vi "Init Events.vi"(8 "error in (no error)":errorcluster, 11 "Main in":refnum<class "Main.lvclass">) -> (0 "error out":errorcluster, 3 "Main out":refnum<class "Main.lvclass">)   [LabVIEW 2019, in "Main.lvclass"]
doc: "Developed by Kevin Thompson\nkevin@thompsonengineering.net\n\nCopyright 2018\nThompson Engineering, LLC"
uses:
  Main.lvclass
  Common/DataTypes/TD Async CmdMsg EventData--cluster.ctl
  Common/DataTypes/UpdateControlValue EvData--cluster.ctl
  DataTypes/ProcessingState--enum.ctl
  DataTypes/ProcessingStateChg EvData--cluster.ctl
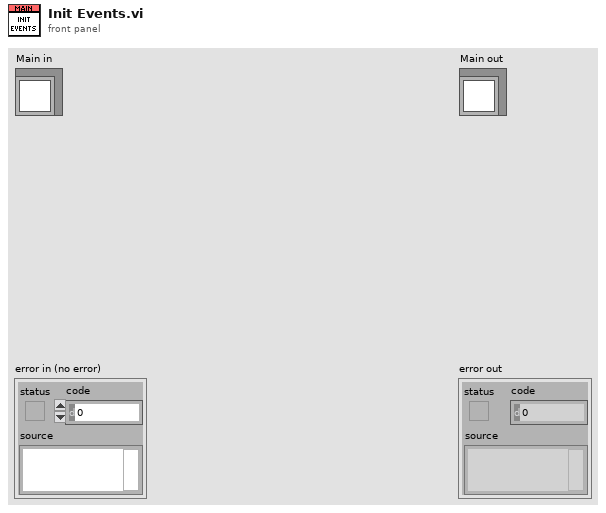
[diagram p1: front panel]
types:
  T1 = typedef "Main.lvclass/ProcessingStateChg EvData--cluster.ctl" = cluster{"Time Stamp":timestamp, "OLD ProcessingState":T2, "NEW ProcessingState":T2}
  T2 = typedef "Main.lvclass/ProcessingState--enum.ctl" = enum16{"Idle", "Starting", "Running", "Done", "Error"}
  T3 = typedef "UpdateControlValue EvData--cluster.ctl" = cluster{"Time Stamp":timestamp, "ControlLabel":string, "vData":variant}
  T4 = typedef "TD Async CmdMsg EventData--cluster.ctl" = cluster{"Time Stamp":timestamp, "CmdMsg":string, "vData":variant}
  T5 = typedef "Main.lvclass/Public Events--cluster.ctl" = cluster{"Main.AsyncCmd Event":refnum<user-event>, "Main.AsyncMsg Event":refnum<user-event>, "stop process":refnum<user-event>, "UpdateControlValue Ev":refnum<user-event>, "ProcessingStateChg Ev":refnum<user-event>}
  T6 = typedef "Main.lvclass/ObjData--cluster.ctl" = cluster{"Settings":T7, "Public Events":T5, "Dependency":T10, "ReadData-placeholder":T11, "VISA-placeholder":refnum<visa-resource-name>, "InverterWaveformsQ":T12, "Application.TerminateProcess Event":refnum<user-event>, "RawDaqDataQ":T13, "MeasSettings":T14, "InverterDataAcqMode":T15, "DAQState Data":T16, "Private Events":T18, "InvWfmsQ-DT":T12, "DPAuxDataQ":T19, "ProcessingState":T2, "InverterInfo":T20, "CurrInverters":T21[], "InverterLUT Dict":T25, "ESR Chart Ref":refnum<vi>, "StoreESR BLine Ref":refnum<vi>, "UseSavedESR BLine Ref":refnum<vi>}
  T7 = typedef "Main.lvclass/Settings--cluster.ctl" = cluster{"Simulation":bool, "Signal scaling":T8[], "ESR scaling":T9[], "num readings to average":i32[], "ESR alarm threshhold (%)":i32[], "UseDummyVrms":bool, "Dummy Vrms":dbl, "Inverter Database File":path, "default Inverter (name)":string[]}
  T8 = typedef "Main.lvclass/Gain control.ctl" = cluster{"Iin ripple gain":dbl, "Iout ripple gain":dbl, "Iout 60Hz gain ":dbl, "Vout 60Hz gain ":dbl, "Iin ripple offest":dbl, "Iout ripple offset":dbl, "Iout 60Hz offset":dbl, "Vout 60Hz offset":dbl}
  T9 = typedef "Main.lvclass/ESR scaling--cluster.ctl" = cluster{"Gain":dbl, "Offset":dbl}
  T10 = typedef "Main.lvclass/Dependency--cluster.ctl" = cluster{"Config":refnum<class "Config.lvclass">, "DAQ":refnum<class "DAQ_Engine.lvclass">, "Log_Engine":refnum<class "Log_Engine.lvclass">}
  T11 = typedef "Main.lvclass/Read Data--cluster.ctl" = cluster{"Data":dbl}
  T12 = typedef "InverterWaveforms--QRef.ctl" = refnum<queue>
  T13 = typedef "RawDAQDataQRef--cluster.ctl" = refnum<queue>
  T14 = typedef "Measurement Config--cluster.ctl" = cluster{"Data Rate 9775":dbl, "Data Rate 9215":dbl, "Samples RMS 9215":u32, "Samples RMS 9775":u32}
  T15 = typedef "Acquisition Mode--cluster.ctl" = enum16{"3phase", "Single"}
  T16 = typedef "DAQ_Engine.lvclass/DAQStateEvData--cluster.ctl" = cluster{"DAQState":T17, "vData":variant}
  T17 = typedef "DAQState--enum.ctl" = enum16{"Unknown", "Stopped", "Running", "Error"}
  T18 = typedef "Main.lvclass/Private Events--cluster.ctl" = cluster{"PrivateAsync Ev":refnum<user-event>}
  T19 = typedef "DataProcAuxDat--Qref.ctl" = refnum<queue>
  T20 = typedef "InverterInfo--cluster.ctl" = cluster{"Inverter ID":string}
  T21 = typedef "Inverter database record v2--cluster.ctl" = cluster{"name":string, "last updated":timestamp, "type":string, "inverter Info":T22, "gain range":T23, "offset range":T24, "gain actual":dbl, "offset actual":dbl, "power level":dbl, "minimum current":dbl, "resistance single phase":dbl, "resistance 3 phase":dbl, "set flag":u16}
  T22 = typedef "inverter info v2--cluster.ctl" = cluster{"manufacturer":string, "model":string, "product":string, "serial":string, "power class":string, "year manf":string}
  T23 = typedef "inverter gain range--cluster.ctl" = cluster{"gain max":dbl, "gain min":dbl, "gain increment":dbl}
  T24 = typedef "inverter offset range--cluster.ctl" = cluster{"offset max":dbl, "offset min":dbl, "offset increment":dbl}
  T25 = typedef "TD Dynamic CVT DVR--ref.ctl" = refnum<data-value>
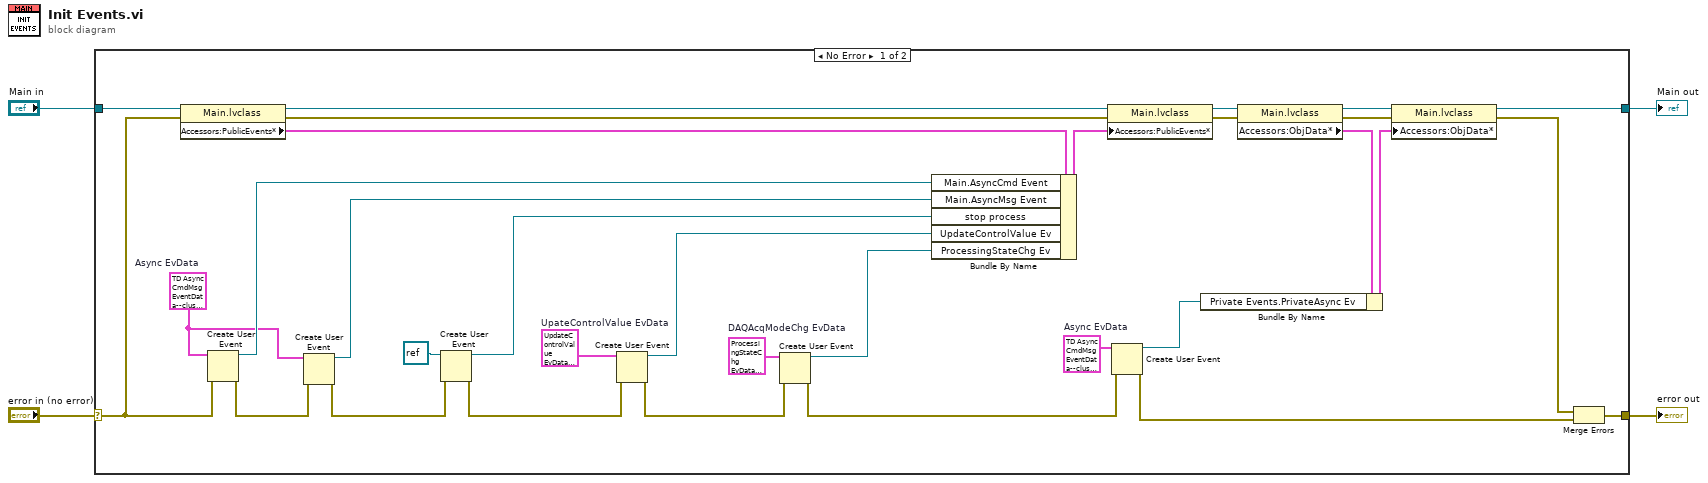
[diagram p0: block diagram]
diagram:
  n1 = case shown="No Error" "error in (no error)" {
    selector: "error in (no error)" -> [w14 w38]
    tunnel: [w12 w38] -> w3
    tunnel: [w10 w37] -> w1
    tunnel: "Main in" -> [w35 w37]
    frame No Error {
      w18 = T1 {"Time Stamp"=timestamp(0 s since 1904-01-01), "OLD ProcessingState"=enum."Idle", "NEW ProcessingState"=enum."Idle"}  # DAQAcqModeChg EvData
      w20 = T3 {"Time Stamp"=timestamp(0 s since 1904-01-01), "ControlLabel"="", "vData"=variant}  # UpateControlValue EvData
      w23 = T4 {"Time Stamp"=timestamp(0 s since 1904-01-01), "CmdMsg"="", "vData"=variant}  # Async EvData
      w26 = T4 {"Time Stamp"=timestamp(0 s since 1904-01-01), "CmdMsg"="", "vData"=variant}  # Async EvData
      n2 = property class="Main.lvclass"(reference=w35, error in=w14) -> (reference out=w34:refnum<class "Main.lvclass">, error out=w13:errorcluster, "Accessors:PublicEvents*"=w33:T5)
      n3 = Create User Event(user event datatype=w26, error in=w14) -> (user event=w29:refnum<user-event>, error out=w28:errorcluster)
      n4 = Create User Event(user event datatype=w26, error in=w28) -> (user event=w25:refnum<user-event>, error out=w27:errorcluster)
      n5 = Create User Event(user event datatype=refnum<notifier> refnum ("notifier out"), error in=w27) -> (user event=w30:refnum<user-event>, error out=w21:errorcluster)
      n6 = Create User Event(user event datatype=w20, error in=w21) -> (user event=w19:refnum<user-event>, error out=w17:errorcluster)
      n7 = Create User Event(user event datatype=w18, error in=w17) -> (user event=w15:refnum<user-event>, error out=w16:errorcluster)
      n8 = Bundle By Name(cluster=w33, "Main.AsyncCmd Event"=w29, "Main.AsyncMsg Event"=w25, "stop process"=w30, "UpdateControlValue Ev"=w19, "ProcessingStateChg Ev"=w15) -> (w32:T5)
      n9 = property class="Main.lvclass"(reference=w34, error in=w13, "Accessors:PublicEvents*"=w32) -> (reference out=w36:refnum<class "Main.lvclass">, error out=w8:errorcluster)
      n10 = Create User Event(user event datatype=w23, error in=w16) -> (user event=w22:refnum<user-event>, error out=w24:errorcluster)
      n11 = property class="Main.lvclass"(reference=w36, error in=w8) -> (reference out=w11:refnum<class "Main.lvclass">, error out=w7:errorcluster, "Accessors:ObjData*"=w5:T6)
      n12 = Bundle By Name(cluster=w5, "Private Events.PrivateAsync Ev"=w22) -> (w9:T6)
      n13 = property class="Main.lvclass"(reference=w11, error in=w7, "Accessors:ObjData*"=w9) -> (reference out=w10:refnum<class "Main.lvclass">, error out=w6:errorcluster)
      n14 = Merge Errors(w6, w24) -> (w12:errorcluster)
    }
    frame Error {
    }
  }
  "error out" <- w3
  "Main out" <- w1
